vi "System Function Item.vi"(11 "rSubPane":refnum<vi>) -> (3 "模块定义":T1)   [LabVIEW 2018, in "MainInterface.lvlib"]
uses:
  MainInterface.lvlib
  ModuleInterface/ModuleDefinition.ctl
  ModuleInterface/FunctionItem.ctl
  ModuleInterface/ModuleInterface.lvlib
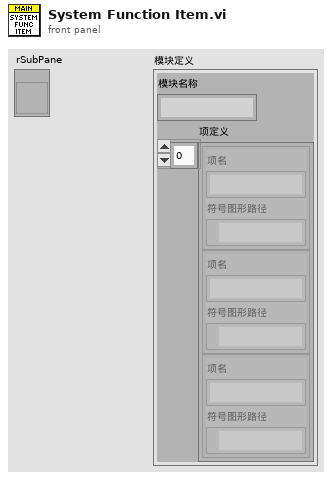
[diagram p1: front panel]
types:
  T1 = typedef "ModuleInterface.lvlib/ModuleDefinition.ctl" = cluster{"模块名称":string, "项定义":T2[]}
  T2 = typedef "ModuleInterface.lvlib/FunctionItem.ctl" = cluster{"项名":string, "符号图形路径":path}
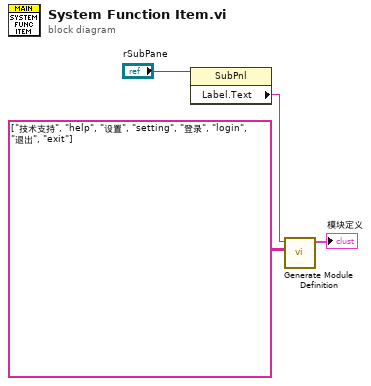
[diagram p0: block diagram]
diagram:
  n1 = property class="SubPnl"(reference="rSubPane") -> ("Label.Text"=w1:string)  [unwired: 1 in, 2 out]
  n2 = call "Generate Module Definition.vi"("数组"=string[][] [["技术支持", "help"], ["设置", "setting"], ["登录", "login"], ["退出", "exit"]], "模块名称"=w1) -> ("模块定义"=→"模块定义":T1)  [unwired: 9 in]
